vi "HEWH Variable Flow Adjustment.vi"(5 "Temp (T) or Flow (F)":bool, 6 "State in":T1, 7 "Variable":dbl, 10 "Target":dbl, 11 "K-Factor (Flow) in":dbl) -> (3 "K-Factor (Flow) out":dbl)   [LabVIEW 2023]
uses:
  Type Definitions/HEWH Purge Draw.ctl
panel:
  in  "Tolerance":dbl=0.25 format="%#_13g"
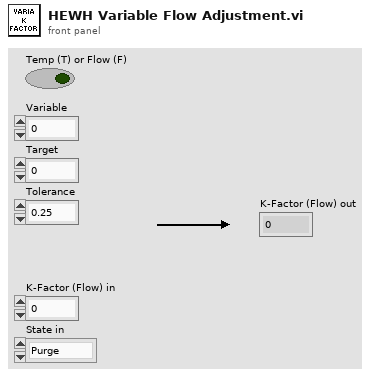
[diagram p1: front panel]
types:
  T1 = typedef "HEWH Purge Draw.ctl" = enum16{"Purge", "Draw"}
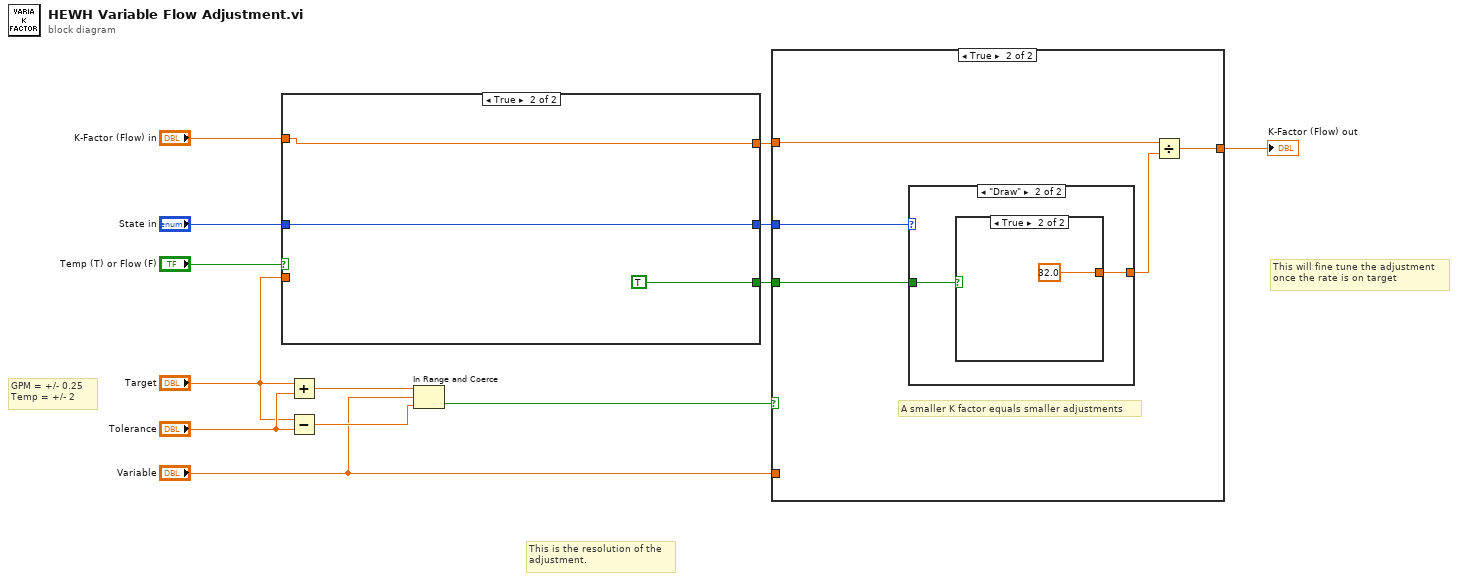
[diagram p0: block diagram]
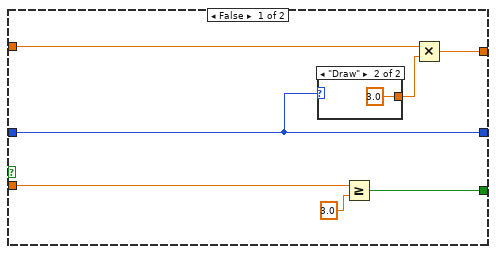
[diagram p2: hidden frame]
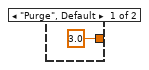
[diagram p3: hidden frame]
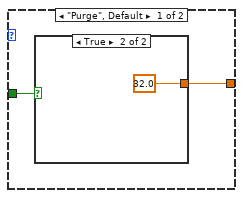
[diagram p5: hidden frame]
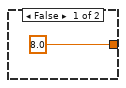
[diagram p6: hidden frame]
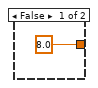
[diagram p7: hidden frame]
diagram:
  # "GPM = +/- 0.25 \nTemp = +/- 2"
  # "This will fine tune the adjustment\nonce the rate is on target"
  # "This is the resolution of the \nadjustment."
  n1 = case shown="True" "Temp (T) or Flow (F)" {
    tunnel: [w19 TRUE] -> w5
    tunnel: "Target" -> [w18 _]
    tunnel: [w16 w24] -> w4
    tunnel: [w14 w23] -> w3
    tunnel: "K-Factor (Flow) in" -> [w15 w24]
    tunnel: "State in" -> [w14 w23]
    frame False {
      n2 = case shown="\"Draw\"" w14 {
        tunnel: [3.0 ("y") 3.0 ("y")] -> w17
        frame "Purge", Default {
        }
        frame "Draw" {
        }
      }
      n3 = Greater Or Equal?(x=w18, y=3.0) -> (x >= y?=w19:bool)
      n4 = Multiply(x=w15, y=w17) -> (x*y=w16:dbl)
    }
    frame True {
    }
  }
  n5 = Add(x="Target", y="Tolerance") -> (x+y=w12:dbl)
  n6 = Subtract(x="Target", y="Tolerance") -> (x-y=w11:dbl)
  n7 = In Range and Coerce(upper limit=w12, x="Variable", lower limit=w11) -> (In Range?=w10:bool)  [unwired: 1 out]
  n8 = case shown="True" w10 {
    tunnel: w4 -> [w26 w31]
    tunnel: [w26 w30] -> w9
    tunnel: w3 -> [_ w28]
    tunnel: "Variable" -> [_ _]
    tunnel: w5 -> [_ w27]
    frame False {
    }
    frame True {
      # "A smaller K factor equals smaller adjustments"
      n9 = case shown="\"Draw\"" w28 {
        tunnel: [w33 w37] -> w29
        tunnel: w27 -> [w32 w36]
        frame "Purge", Default {
          n10 = case shown="True" w32 {
            tunnel: [8.0 ("y") 32.0 ("y")] -> w33
            frame False {
            }
            frame True {
            }
          }
        }
        frame "Draw" {
          n11 = case shown="True" w36 {
            tunnel: [8.0 ("y") 32.0 ("y")] -> w37
            frame False {
            }
            frame True {
            }
          }
        }
      }
      n12 = Divide(x=w31, y=w29) -> (x/y=w30:dbl)
    }
  }
  "K-Factor (Flow) out" <- w9
